vi "oa_Calculate Vector for Given Orders (N Channel)s.vi"(0 "resampled signal":cluster{"r0":dbl, "dr":dbl, "Y":dbl[]}[](array[cluster]) {"r0" format="%.2p"; "dr" format="%.2p"; "Y" format="%.2f"}, 1 "reset? (True)":bool=TRUE, 5 "orders to compensate":dbl[](array[numeric])=[1.0] format="%.2f", 7 "slow roll vectors":cdb[][](array[numeric]) format="%.2f", 9 "interpolated pulse positions":dbl[](array[numeric]) format="%.2f", 11 "error out in":errorcluster) -> (3 "reset out":bool=TRUE, 6 "orders out":dbl[](array[numeric]) min=0.0 max=127.0 format="%.2f", 8 "slow roll vectors":cdb[][](array[numeric]) format="%.2f", 15 "error out":errorcluster)   [LabVIEW 2017, in "SoundVib_RefDataProcess.lvlib"]
uses:
  <vilib>/addons/Sound and Vibration/Order Analysis/Referece Data Processing/SoundVib_RefDataProcess.lvlib
  <vilib>/addons/Sound and Vibration/Order Analysis/Resample Order Tracking/OAT Order Magnitude and Phase (Even Angle Signal, N Channels).vi
  <vilib>/addons/Sound and Vibration/Order Analysis/Resample Order Tracking/SoundVib_OrderTracking.lvlib
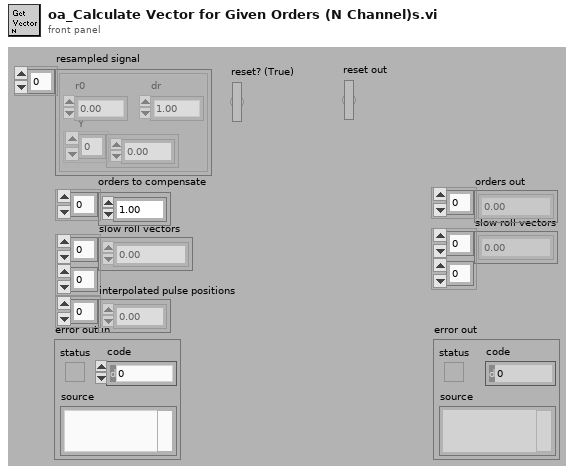
[diagram p1: front panel]
types:
  T1 = cluster{"dB on? (T)":bool, "unwrap phase? (T)":bool, "unit in degree? (T)":bool}
  T2 = typedef "svc_Resampled Channel Info.ctl" = cluster{"channel name":string, "description":string, " channel info":T3}
  T3 = typedef "svc_Channel Info.ctl" = cluster{"sensor sensitivity":dbl, "engineering units":T4, "dB reference":dbl, "custom label":string, "weighting filter":T5, "pregain":dbl}
  T4 = typedef "svc_Engineering Units Text Ring.ctl" = u16
  T5 = typedef "svc_Weighting Filter Text Ring.ctl" = u16
  T6 = cluster{"interpolated pulse positions":dbl[], dbl}
  T7 = cluster{"time/rev/rpm":dbl[], "magnitude":dbl[]}[][]
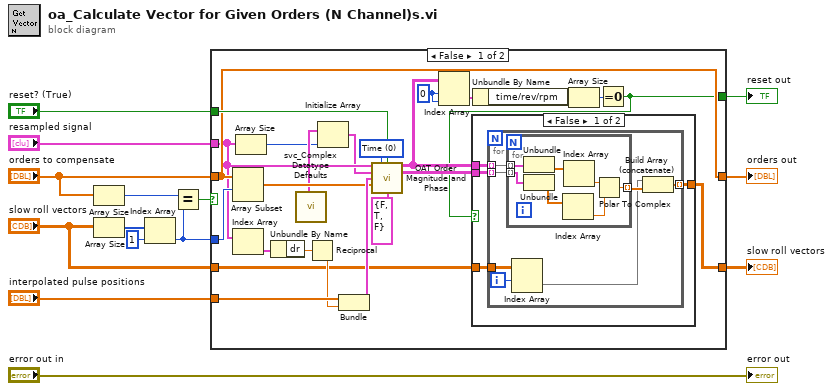
[diagram p0: block diagram]
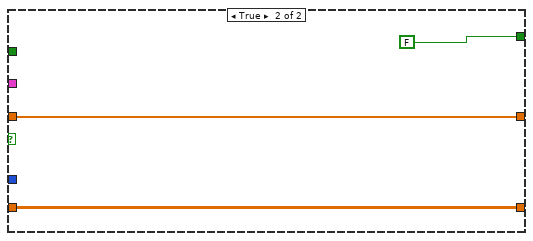
[diagram p3: hidden frame]
diagram:
  n1 = Array Size(array="orders to compensate") -> (size(s)=w12:i32)
  n2 = Array Size(array="slow roll vectors") -> (size(s)=w14:i32[])
  n3 = Index Array(array=w14, index=1) -> (element=w4:i32)
  n4 = Equal?(x=w12, y=w4) -> (x = y?=w11:bool)
  n5 = case shown="False" w11 {
    tunnel: "slow roll vectors" -> [w27 w60]
    tunnel: [w26 w60] -> w9
    tunnel: "orders to compensate" -> [w29 w59]
    tunnel: [w29 w59] -> w7
    tunnel: "resampled signal" -> [w18 _]
    tunnel: w4 -> [w38 _]
    tunnel: "interpolated pulse positions" -> [w37 _]
    tunnel: "reset? (True)" -> [w31 _]
    tunnel: [w20 FALSE] -> w1
    frame False {
      w24 = 0 ("index (row)")
      w32 = u16 0 items=["Time", "Revolution", "RPM"] ("X axis selection")
      n6 = Array Subset(array=w29, index=w38) -> (w19:dbl[])  [unwired: 1 in]
      n7 = Index Array(array=w18) -> (element=w36:cluster{"r0":dbl, "dr":dbl, "Y":dbl[]})  [unwired: 1 in]
      n8 = Array Size(array=w18) -> (size(s)=w16:i32)
      n9 = Unbundle By Name(w36) -> ("dr"=w35:dbl)
      n10 = call <vilib>:"svc_Complex Datatype Defaults.vi"() -> ("resampled channel info"=w17:T2)  [unwired: 11 in, 8 out]
      n11 = Reciprocal(x=w35) -> (1/x=w34:dbl)
      n12 = Initialize Array(w17, w16) -> (w15:T2[])
      n13 = Bundle("interpolated pulse positions"=w37, w34) -> (w33:T6)  [unwired: 1 in]
      n14 = call-poly <vilib>:"OAT Order Magnitude and Phase.vi"("even-angle signals"=w18, "x-axis selection"=w32, "reset? (F)"=w31, "even-angle channel info"=w15, "even-angle position info"=w33, "orders to compute (1.0)"=w19, "view"=T1 {"dB on? (T)"=FALSE, "unwrap phase? (T)"=TRUE, "unit in degree? (T)"=FALSE}) -> ("magnitudes [RMS]"=w25:T7, "phases [phase lag]"=w28:cluster{"time/rev/rpm":dbl[], "phase":dbl[]}[][])  [unwired: 3 in, 4 out]
      n15 = Index Array(array=w25, index (row)=w24, index (col)=w24) -> (element=w23:cluster{"time/rev/rpm":dbl[], "magnitude":dbl[]})
      n16 = Unbundle By Name(w23) -> ("time/rev/rpm"=w22:dbl[])
      n17 = Array Size(array=w22) -> (size(s)=w21:i32)
      n18 = Equal To 0?(x=w21) -> (x = 0?=w20:bool)
      n19 = case shown="False" w20 {
        tunnel: w28 -> [w42 _]
        tunnel: w27 -> [w41 w57]
        tunnel: [w40 w57] -> w26
        tunnel: w25 -> [w39 _]
        frame False {
          n20 = for {
            tunnel: w39 -> [w47] mode=indexing
            tunnel: w42 -> [w46] mode=indexing
            tunnel: w41 -> [w49]
            tunnel: [w43] -> w40 mode=indexing
            i -> [w48]
            n21 = for {
              tunnel: w47 -> [w56] mode=indexing
              tunnel: w46 -> [w55] mode=indexing
              tunnel: [w50] -> w45 mode=indexing
              n22 = Unbundle(w56) -> ("magnitude"=w52:dbl[])  [unwired: 1 out]
              n23 = Unbundle(w55) -> ("phase"=w51:dbl[])  [unwired: 1 out]
              n24 = Index Array(array=w51) -> (element=w53:dbl)  [unwired: 1 in]
              n25 = Index Array(array=w52) -> (element=w54:dbl)  [unwired: 1 in]
              n26 = Polar To Complex(1:w53, 2:w54) -> (0:w50:cdb)
            }
            n27 = Index Array(array=w49, index (row)=w48) -> (element=w44:cdb[])  [unwired: 1 in]
            n28 = Build Array (concatenate)(w44, w45) -> (w43:cdb[])
          }
        }
        frame True {
        }
      }
    }
    frame True {
    }
  }
  "slow roll vectors" <- w9
  "orders out" <- w7
  "reset out" <- w1
  "error out" <- "error out in"
